vi "Initialize.vi"(8 "error in (no error)":errorcluster, 11 "ProjectBase in":refnum<class "Project.lvclass">) -> (0 "error out":errorcluster, 3 "ProjectBase out":refnum<class "Project.lvclass">)   [LabVIEW 2015, in "Project.lvclass"]
uses:
  Project.lvclass
  Step.lvclass
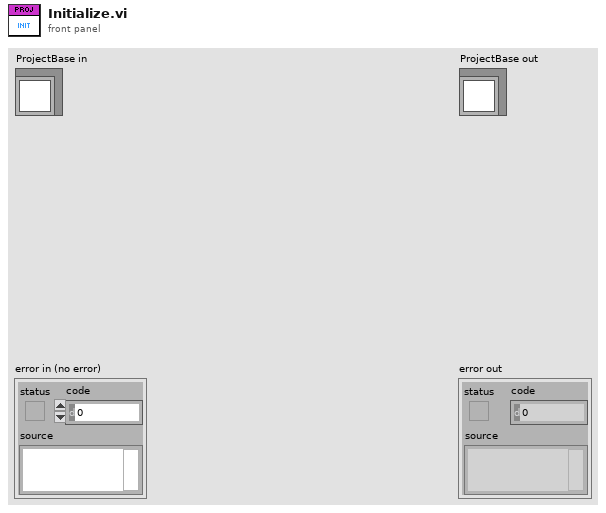
[diagram p1: front panel]
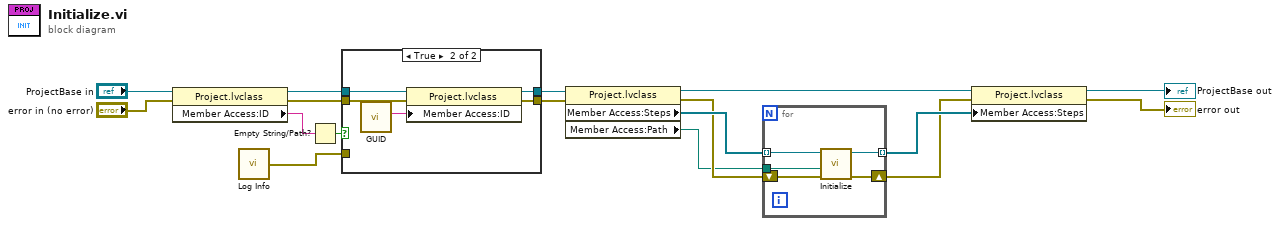
[diagram p0: block diagram]
diagram:
  n1 = property class="Project.lvclass"(reference="ProjectBase in", error in="error in (no error)") -> (reference out=w15:refnum<class "Project.lvclass">, error out=w14:errorcluster, "Member Access:ID"=w13:string)
  n2 = call "Log Info.vi"() -> ("error out"=w1:errorcluster)  [unwired: 5 in]
  n3 = Empty String/Path?(string/path=w13) -> (empty?=w12:bool)
  n4 = case shown="True" w12 {
    tunnel: [w18 w23] -> w10
    tunnel: [w19 w22] -> w11
    tunnel: w15 -> [w19 w21]
    tunnel: w14 -> [w18 w20]
    tunnel: w1 -> [_ _]
    frame False {
    }
    frame True {
      n5 = call "GUID.vi"() -> ("GUID"=w24:string)  [unwired: 10 in, 1 out]
      n6 = property class="Project.lvclass"(reference=w21, error in=w20, "Member Access:ID"=w24) -> (reference out=w22:refnum<class "Project.lvclass">, error out=w23:errorcluster)
    }
  }
  n7 = property class="Project.lvclass"(reference=w11, error in=w10) -> (reference out=w5:refnum<class "Project.lvclass">, error out=w6:errorcluster, "Member Access:Steps"=w7:refnum<class "Step.lvclass">[], "Member Access:Path"=w2:path)
  n8 = for {
    tunnel: w7 -> [w29] mode=indexing
    tunnel: [w27] -> w4 mode=indexing
    shift-right: [w26] -> w3
    shift-left: w6 -> [w28]
    tunnel: w2 -> [w25]
    n9 = call-dynamic "Initialize.vi"("error in (no error)"=w28, "Project Path"=w25, "Step in"=w29) -> ("error out"=w26:errorcluster, "Step out"=w27:refnum<class "Step.lvclass">)  [unwired: 7 in]
  }
  n10 = property class="Project.lvclass"(reference=w5, error in=w3, "Member Access:Steps"=w4) -> (reference out=→"ProjectBase out":refnum<class "Project.lvclass">, error out=→"error out":errorcluster)
